vi "Template jsObject.vi"(8 "error in (no error)":errorcluster, 9 "Template Record (empty)":T1, 10 "Template jsObject Name (\"\")":string, 11 "Previous String (\"\")":string) -> (0 "error out":errorcluster, 2 "Template jsObject":string, 3 "Template jsObject Definition":string)   [LabVIEW 2011]
uses:
  Template Record.ctl
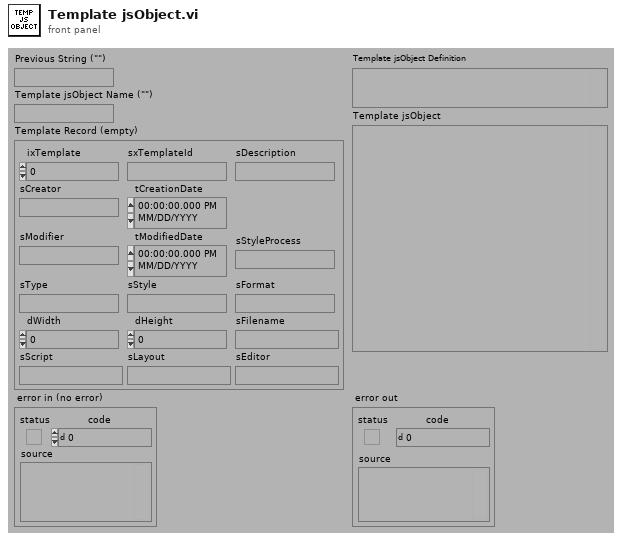
[diagram p1: front panel]
types:
  T1 = typedef "Template Record.ctl" = cluster{"ixTemplate":i32, "sxTemplateId":string, "sDescription":string, "sCreator":string, "tCreationDate":timestamp, "sModifier":string, "tModifiedDate":timestamp, "sType":string, "sStyle":string, "sFormat":string, "dWidth":dbl, "dHeight":dbl, "sFilename":string, "sScript":string, "sLayout":string, "sEditor":string, "sStyleProcess":string}
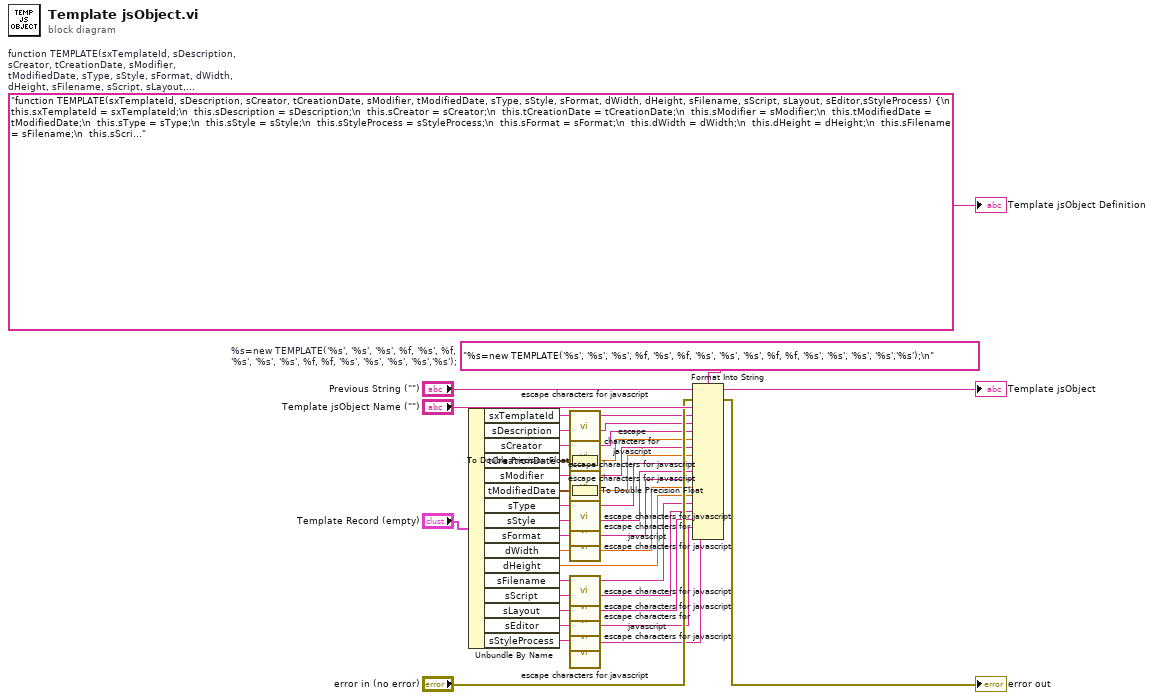
[diagram p0: block diagram]
diagram:
  w31 = "function TEMPLATE(sxTemplateId, sDescription, sCreator, tCreationDate, sModifier, tModifiedDate, sType, sStyle, sFormat, dWidth, dHeight, sFilename, sScript, sLayout, sEditor,sStyleProcess) {\n  this.sxTemplateId = sxTemplateId;\n  this.sDescription = sDescription;\n  this.sCreator = sCreator;\n  this.tCreationDate = tCreationDate;\n  this.sModifier = sModifier;\n  this.tModifiedDate = tModifiedDate;\n  this.sType = sType;\n  this.sStyle = sStyle;\n  this.sStyleProcess = sStyleProcess;\n  this.sFormat = sFormat;\n  this.dWidth = dWidth;\n  this.dHeight = dHeight;\n  this.sFilename = sFilename;\n  this.sScript = sScript;\n  this.sLayout = sLayout;\n  this.sEditor = sEditor;\n}"  # function TEMPLATE(sxTemplateId, sDescription, sCreator, tCreationDate, sModifier, tModifiedDate, sType, sStyle, sFormat, dWidth, dHeight, sFilename, sScript, sLayout, sEditor,sStyleProcess) {   this.sxTemplateId = sxTemplateId;   this.sDescription = sDescription;   this.sCreator = sCreator;   this.tCreationDate = tCreationDate;   this.sModifier = sModifier;   this.tModifiedDate = tModifiedDate;   this.sType = sType;   this.sStyle = sStyle;   this.sStyleProcess = sStyleProcess;   this.sFormat = sFormat;   this.dWidth = dWidth;   this.dHeight = dHeight;   this.sFilename = sFilename;   this.sScript = sScript;   this.sLayout = sLayout;   this.sEditor = sEditor; }
  w38 = "%s=new TEMPLATE('%s', '%s', '%s', %f, '%s', %f, '%s', '%s', '%s', %f, %f, '%s', '%s', '%s', '%s','%s');\n"  # %s=new TEMPLATE('%s', '%s', '%s', %f, '%s', %f, '%s', '%s', '%s', %f, %f, '%s', '%s', '%s', '%s','%s');
  n1 = Unbundle By Name("Template Record (empty)") -> ("sxTemplateId"=w30:string, "sDescription"=w29:string, "sCreator"=w27:string, "tCreationDate"=w28:timestamp, "sModifier"=w3:string, "tModifiedDate"=w26:timestamp, "sType"=w23:string, "sStyle"=w24:string, "sFormat"=w25:string, "dWidth"=w9:dbl, "dHeight"=w8:dbl, "sFilename"=w19:string, "sScript"=w20:string, "sLayout"=w21:string, "sEditor"=w22:string, "sStyleProcess"=w2:string)
  n2 = call "escape characters for javascript.vi"("String (\"\")"=w30) -> ("escaped String"=w18:string)  [unwired: 4 out]
  n3 = call "escape characters for javascript.vi"("String (\"\")"=w29) -> ("escaped String"=w17:string)  [unwired: 4 out]
  n4 = call "escape characters for javascript.vi"("String (\"\")"=w27) -> ("escaped String"=w16:string)  [unwired: 4 out]
  n5 = To Double Precision Float(number=w28) -> (double precision float=w15:dbl)
  n6 = call "escape characters for javascript.vi"("String (\"\")"=w3) -> ("escaped String"=w14:string)  [unwired: 4 out]
  n7 = To Double Precision Float(number=w26) -> (double precision float=w13:dbl)
  n8 = call "escape characters for javascript.vi"("String (\"\")"=w23) -> ("escaped String"=w12:string)  [unwired: 4 out]
  n9 = call "escape characters for javascript.vi"("String (\"\")"=w24) -> ("escaped String"=w11:string)  [unwired: 4 out]
  n10 = call "escape characters for javascript.vi"("String (\"\")"=w25) -> ("escaped String"=w10:string)  [unwired: 4 out]
  n11 = call "escape characters for javascript.vi"("String (\"\")"=w19) -> ("escaped String"=w7:string)  [unwired: 4 out]
  n12 = call "escape characters for javascript.vi"("String (\"\")"=w20) -> ("escaped String"=w6:string)  [unwired: 4 out]
  n13 = call "escape characters for javascript.vi"("String (\"\")"=w21) -> ("escaped String"=w5:string)  [unwired: 4 out]
  n14 = call "escape characters for javascript.vi"("String (\"\")"=w22) -> ("escaped String"=w4:string)  [unwired: 4 out]
  n15 = call "escape characters for javascript.vi"("String (\"\")"=w2) -> ("escaped String"=w1:string)  [unwired: 4 out]
  n16 = Format Into String(format string=w38, initial string="Previous String (\"\")", error in="error in (no error)", "Template jsObject Name (\"\")", w18, w17, w16, w15, w14, w13, w12, w11, w10, w9, w8, w7, w6, w5, w4, w1) -> (resulting string=→"Template jsObject":string, error out=→"error out":errorcluster)
  "Template jsObject Definition" <- w31
